vi "Receive Value Change Event.vi"(8 "error in (no error)":errorcluster, 10 "ValueChangeMsg":refnum<class "ValueChangeMsg.lvclass">, 11 "Car Position Simulation View Definition In":refnum<class "Car Position Simulation View Definition.lvclass">) -> (0 "error out":errorcluster, 3 "Car Position Simulation View Definition Out":refnum<class "Car Position Simulation View Definition.lvclass">)   [LabVIEW 2019, in "Car Position Simulation View Definition.lvclass"]
doc: "<License>\nCopyright © 2017 Composed Systems, LLC | All rights reserved\nwww.composed.io\n\nAuthor: Ethan Stern <ethan.stern@composed.io>\n\nThis software is provided \"AS IS\" WITHOUT WARRANTIES, either express or implied, AND IS FOR EDUCATIONAL PURPOSES ONLY.\n</License>"
uses:
  <vilib>/gpm_packages/@cs/Car-wash/Source/Car Position Simulation View Definition/Car Position Simulation View Definition/Car Position Simulation View Definition.lvclass
  <vilib>/gpm_packages/@cs/mva-viewable/Source/ActorEvents/IEventAggregator Messages/ValueChangeMsg/ValueChangeMsg.lvclass
  <vilib>/gpm_packages/@cs/mva-viewable/Source/IViewable/IViewable/IViewable.lvclass
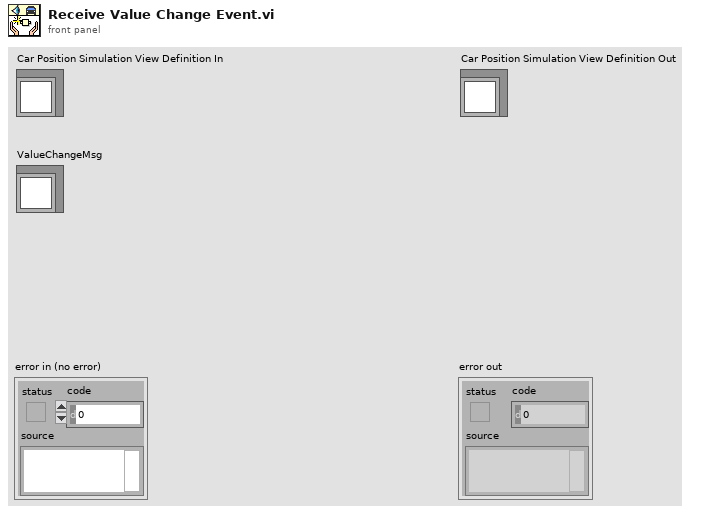
[diagram p1: front panel]
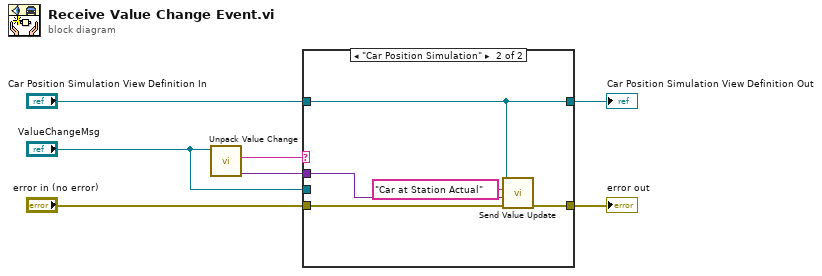
[diagram p0: block diagram]
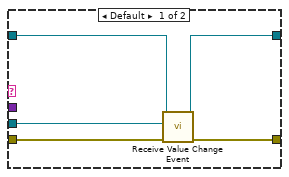
[diagram p2: hidden frame]
diagram:
  n1 = call <vilib>:"Unpack Value Change.vi"("ValueChangeMsg"="ValueChangeMsg") -> ("New Value"=w1:variant, "Control Label"=w2:string)  [unwired: 6 in, 3 out]
  n2 = case shown="\"Car Position Simulation\"" w2 {
    tunnel: [w12 w16] -> w7
    tunnel: [w11 w17] -> w6
    tunnel: "error in (no error)" -> [w10 w14]
    tunnel: "Car Position Simulation View Definition In" -> [w9 w17]
    tunnel: "ValueChangeMsg" -> [w8 _]
    tunnel: w1 -> [_ w13]
    frame Default {
      n3 = call-parent "Receive Value Change Event.vi"("error in (no error)"=w10, "ValueChangeMsg"=w8, "IViewable In"=w9) -> ("error out"=w12:errorcluster, "IViewable Out"=w11:refnum<class "Car Position Simulation View Definition.lvclass">)  [unwired: 7 in]
    }
    frame "Car Position Simulation" {
      n4 = call-dynamic "Send Value Update.vi"("error in (no error)"=w14, "Value"=w13, "Datum Name"="Car at Station Actual", "IViewable in"=w17) -> ("error out"=w16:errorcluster)  [unwired: 7 in]
    }
  }
  "error out" <- w7
  "Car Position Simulation View Definition Out" <- w6
